vi "closeDateImages.vi"(11 "data":T1) -> (0 "error out":errorcluster)   [LabVIEW 2020, in "MagAnalysis_Online.lvclass"]
uses:
  MagAnalysis_Online.lvclass
  analysis_data_typdef.ctl
  IMAQ Image.ctl
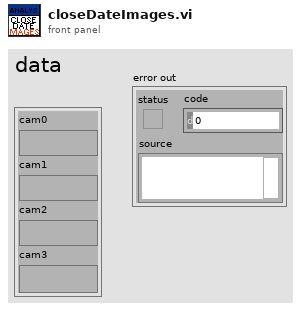
[diagram p1: front panel]
types:
  T1 = typedef "MagAnalysis_Online.lvclass/analysis_data_typdef.ctl" = cluster{"cam0":T2, "cam1":T2, "cam2":T2, "cam3":T2}
  T2 = typedef "IMAQ Image.ctl" = refnum<image>
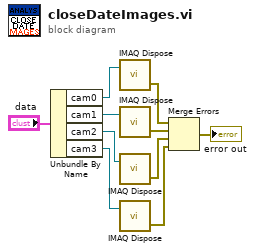
[diagram p0: block diagram]
diagram:
  n1 = Unbundle By Name("data") -> ("cam0"=w2:T2, "cam1"=w3:T2, "cam2"=w4:T2, "cam3"=w5:T2)
  n2 = call "IMAQ Dispose"("Image"=w2) -> ("error out"=w6:errorcluster)  [unwired: 5 in]
  n3 = call "IMAQ Dispose"("Image"=w3) -> ("error out"=w7:errorcluster)  [unwired: 5 in]
  n4 = call "IMAQ Dispose"("Image"=w4) -> ("error out"=w8:errorcluster)  [unwired: 5 in]
  n5 = call "IMAQ Dispose"("Image"=w5) -> ("error out"=w9:errorcluster)  [unwired: 5 in]
  n6 = Merge Errors(w6, w7, w8, w9) -> (→"error out":errorcluster)
